vi "LVAPT_Git_Menu_Hierachy.vi"(11 "ProjectPath":path) -> (3 "Array":T1[](array[typedef]))   [LabVIEW 2019]
uses:
  <resource>/Framework/Providers/API/mxLvMenuItem.ctl
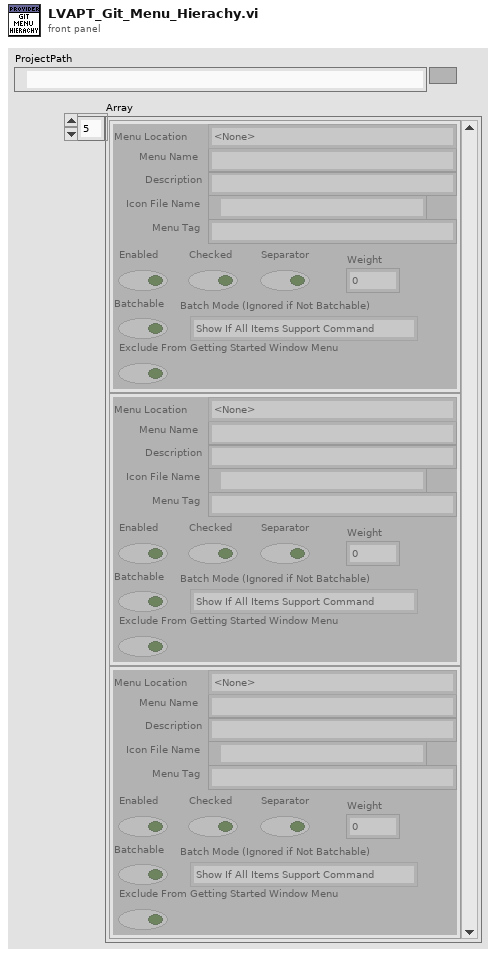
[diagram p1: front panel]
types:
  T1 = typedef "mxLvMenuItem.ctl" = cluster{"Menu Name":string, "Description":string, "Icon File Name":path, "Menu Tag":string, "Enabled":bool, "Checked":bool, "Separator":bool, "Batchable":bool, "Weight":i32, "Batch Mode (Ignored if Not Batchable)":enum32{"Show If All Items Support Command", "Show If Any Items Support Command"}, "Menu Location":enum32{"<None>", "Project", "Project / Build Specifications", "Tools", "Tools / Source Control", "Tools / Real-Time Module", "Help"}, "Exclude From Getting Started Window Menu":bool}
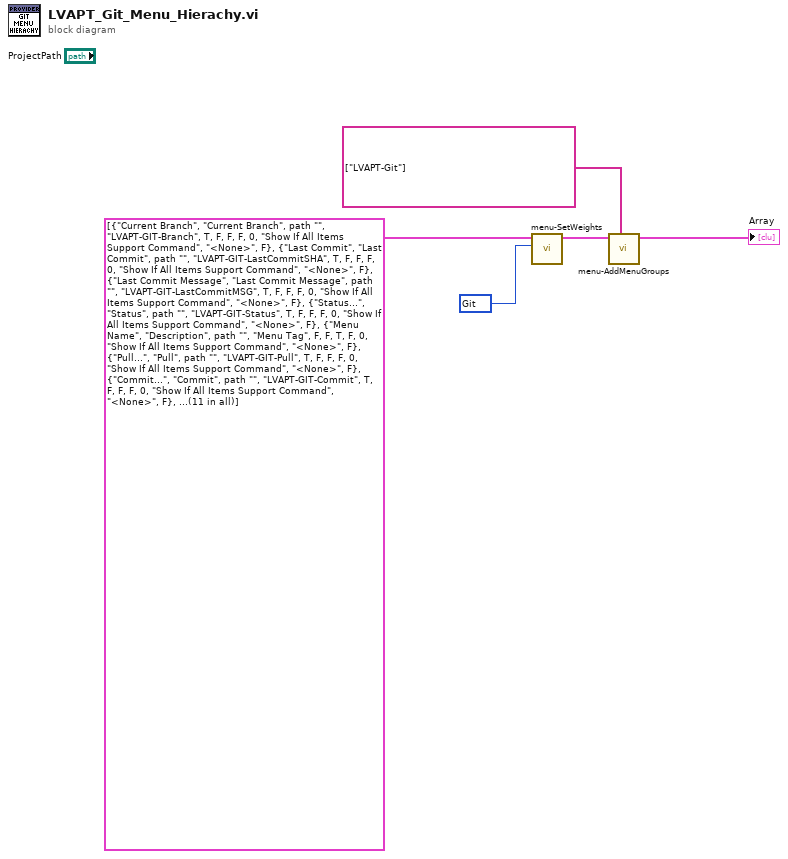
[diagram p0: block diagram]
diagram:
  w2 = u32 4529000 items=["DEV_Env"=4520000, "<2>"=1, "<3>"=2, "SystemProviders"=4523000, "<5>"=4, "<6>"=5, "ToolProviders"=4527000, "Development Tools"=4528000, "Git"=4529000] ("Ring")
  n1 = call "menu-SetWeights.vi"("Start"=w2, "Array in"=T1[] [{"Menu Name"="Current Branch", "Description"="Current Branch", "Icon File Name"=path "", "Menu Tag"="LVAPT-GIT-Branch", "Enabled"=TRUE, "Checked"=FALSE, "Separator"=FALSE, "Batchable"=FALSE, "Weight"=0, "Batch Mode (Ignored if Not Batchable)"=enum."Show If All Items Support Command", "Menu Location"=enum."<None>", "Exclude From Getting Started Window Menu"=FALSE}, {"Menu Name"="Last Commit", "Description"="Last Commit", "Icon File Name"=path "", "Menu Tag"="LVAPT-GIT-LastCommitSHA", "Enabled"=TRUE, "Checked"=FALSE, "Separator"=FALSE, "Batchable"=FALSE, "Weight"=0, "Batch Mode (Ignored if Not Batchable)"=enum."Show If All Items Support Command", "Menu Location"=enum."<None>", "Exclude From Getting Started Window Menu"=FALSE}, {"Menu Name"="Last Commit Message", "Description"="Last Commit Message", "Icon File Name"=path "", "Menu Tag"="LVAPT-GIT-LastCommitMSG", "Enabled"=TRUE, "Checked"=FALSE, "Separator"=FALSE, "Batchable"=FALSE, "Weight"=0, "Batch Mode (Ignored if Not Batchable)"=enum."Show If All Items Support Command", "Menu Location"=enum."<None>", "Exclude From Getting Started Window Menu"=FALSE}, {"Menu Name"="Status...", "Description"="Status", "Icon File Name"=path "", "Menu Tag"="LVAPT-GIT-Status", "Enabled"=TRUE, "Checked"=FALSE, "Separator"=FALSE, "Batchable"=FALSE, "Weight"=0, "Batch Mode (Ignored if Not Batchable)"=enum."Show If All Items Support Command", "Menu Location"=enum."<None>", "Exclude From Getting Started Window Menu"=FALSE}, {"Menu Name"="Menu Name", "Description"="Description", "Icon File Name"=path "", "Menu Tag"="Menu Tag", "Enabled"=FALSE, "Checked"=FALSE, "Separator"=TRUE, "Batchable"=FALSE, "Weight"=0, "Batch Mode (Ignored if Not Batchable)"=enum."Show If All Items Support Command", "Menu Location"=enum."<None>", "Exclude From Getting Started Window Menu"=FALSE}, {"Menu Name"="Pull...", "Description"="Pull", "Icon File Name"=path "", "Menu Tag"="LVAPT-GIT-Pull", "Enabled"=TRUE, "Checked"=FALSE, "Separator"=FALSE, "Batchable"=FALSE, "Weight"=0, "Batch Mode (Ignored if Not Batchable)"=enum."Show If All Items Support Command", "Menu Location"=enum."<None>", "Exclude From Getting Started Window Menu"=FALSE}, {"Menu Name"="Commit...", "Description"="Commit", "Icon File Name"=path "", "Menu Tag"="LVAPT-GIT-Commit", "Enabled"=TRUE, "Checked"=FALSE, "Separator"=FALSE, "Batchable"=FALSE, "Weight"=0, "Batch Mode (Ignored if Not Batchable)"=enum."Show If All Items Support Command", "Menu Location"=enum."<None>", "Exclude From Getting Started Window Menu"=FALSE}, {"Menu Name"="Push...", "Description"="Push", "Icon File Name"=path "", "Menu Tag"="LVAPT-GIT-Push", "Enabled"=TRUE, "Checked"=FALSE, "Separator"=FALSE, "Batchable"=FALSE, "Weight"=0, "Batch Mode (Ignored if Not Batchable)"=enum."Show If All Items Support Command", "Menu Location"=enum."<None>", "Exclude From Getting Started Window Menu"=FALSE}, {"Menu Name"="Menu Name", "Description"="Description", "Icon File Name"=path "", "Menu Tag"="Menu Tag", "Enabled"=FALSE, "Checked"=FALSE, "Separator"=TRUE, "Batchable"=FALSE, "Weight"=0, "Batch Mode (Ignored if Not Batchable)"=enum."Show If All Items Support Command", "Menu Location"=enum."<None>", "Exclude From Getting Started Window Menu"=FALSE}, {"Menu Name"="Switch To Daily Branch", "Description"="Switch To Daily Branch", "Icon File Name"=path "", "Menu Tag"="LVAPT-GIT-SwitchToDailyBranch", "Enabled"=TRUE, "Checked"=FALSE, "Separator"=FALSE, "Batchable"=FALSE, "Weight"=0, "Batch Mode (Ignored if Not Batchable)"=enum."Show If All Items Support Command", "Menu Location"=enum."<None>", "Exclude From Getting Started Window Menu"=FALSE}, {"Menu Name"="Leave Daily Branch", "Description"="Leave Daily Branch", "Icon File Name"=path "", "Menu Tag"="LVAPT-GIT-LeaveDailyBranch", "Enabled"=TRUE, "Checked"=FALSE, "Separator"=FALSE, "Batchable"=FALSE, "Weight"=0, "Batch Mode (Ignored if Not Batchable)"=enum."Show If All Items Support Command", "Menu Location"=enum."<None>", "Exclude From Getting Started Window Menu"=FALSE}] ("Array")) -> ("Array out"=w3:T1[])  [unwired: 9 in]
  n2 = call "menu-AddMenuGroups.vi"("Menu Name"=string[] ["LVAPT-Git"], "element"=w3) -> ("Array"=→"Array":T1[])  [unwired: 9 in]
